vi "Logger File Create.vi"(8 "error in":errorcluster, 9 "Test Stand Name":string, 10 "Project Base Path":path, 11 "UI Logger in":refnum<class "UI Logger.lvclass">) -> (0 "error out":errorcluster, 3 "UI Logger out":refnum<class "UI Logger.lvclass">)   [LabVIEW 2019, in "TS Framework.lvlib" / "UI Logger.lvclass"]
uses:
  UI Logger.lvclass
  Logger/Logger.lvclass
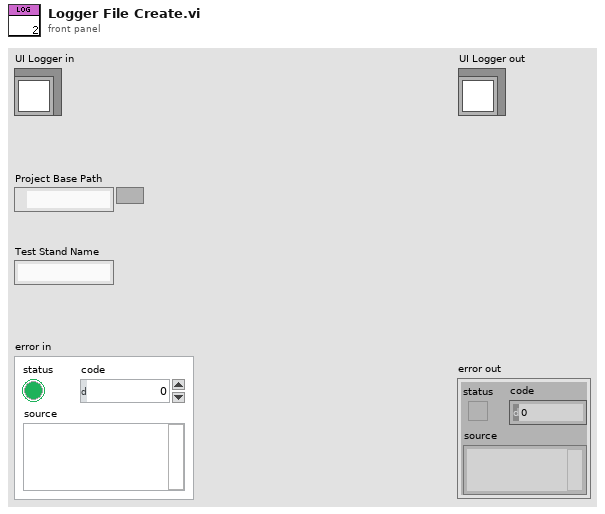
[diagram p1: front panel]
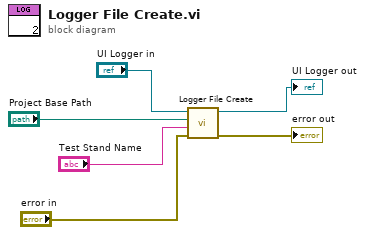
[diagram p0: block diagram]
diagram:
  n1 = call-parent "Logger File Create.vi"("error in"="error in", "Test Stand Name"="Test Stand Name", "Project Base Path"="Project Base Path", "Logger in"="UI Logger in") -> ("error out"=→"error out":errorcluster, "Logger out"=→"UI Logger out":refnum<class "UI Logger.lvclass">)  [unwired: 6 in]
